vi "StateMachineExample.vi"() -> ()   [LabVIEW 2018]
doc: "Use this template to build a simple state machine design pattern. Each state executes code and determines which state to transition to."
panel:
  out "Data Ex out":T1
  in  "Data Ex":T1
  out "x .or. y?":bool
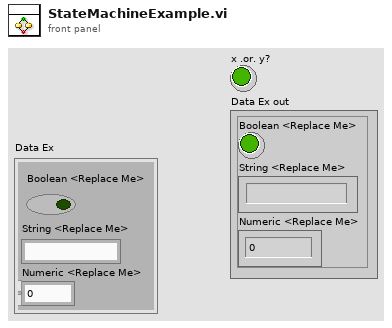
[diagram p1: front panel]
types:
  T1 = cluster{"Boolean <Replace Me>":bool, "String <Replace Me>":string, "Numeric <Replace Me>":dbl}
  T2 = enum16{"Initialize", "State 1", "State 2", "Exit"}
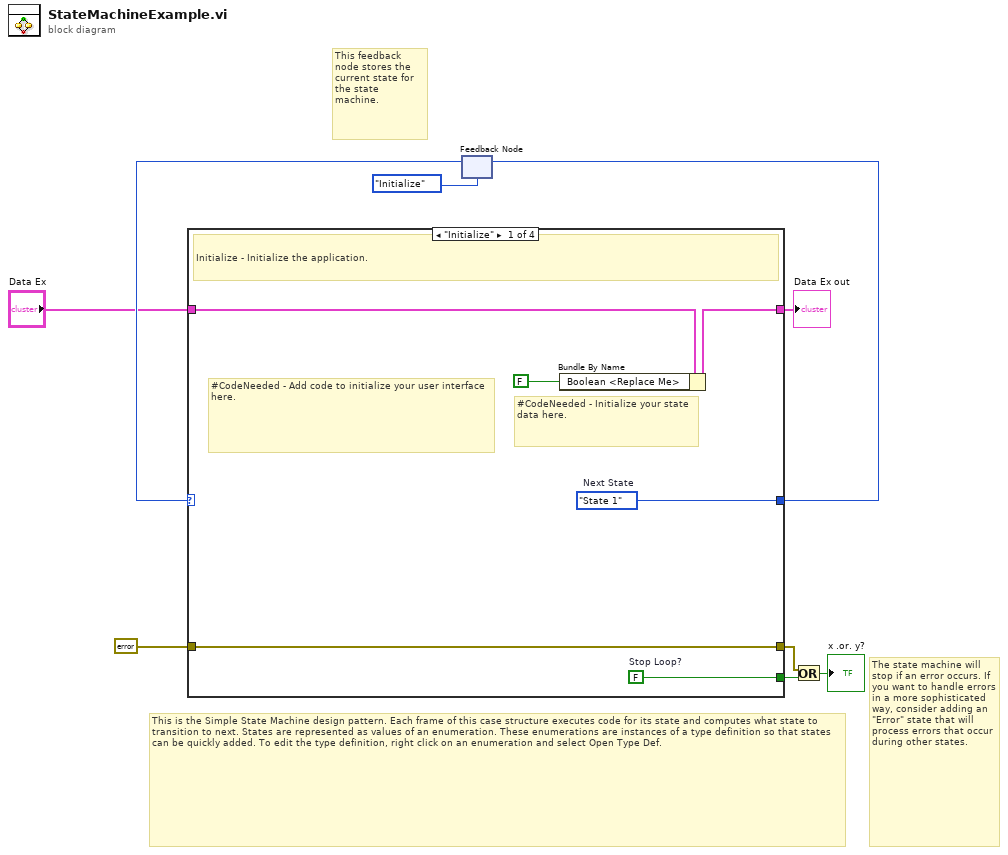
[diagram p0: block diagram]
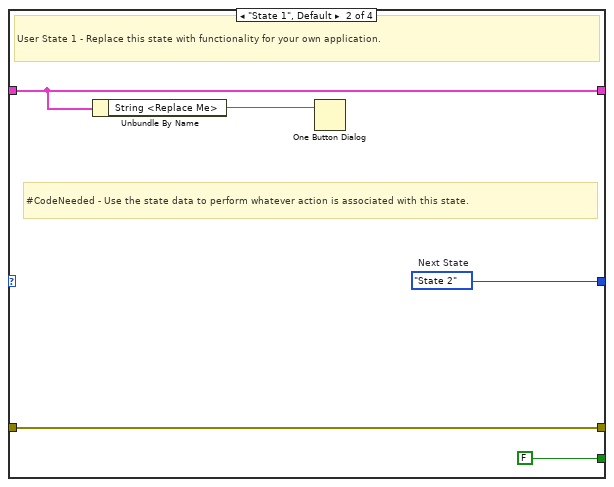
[diagram p2: hidden frame]
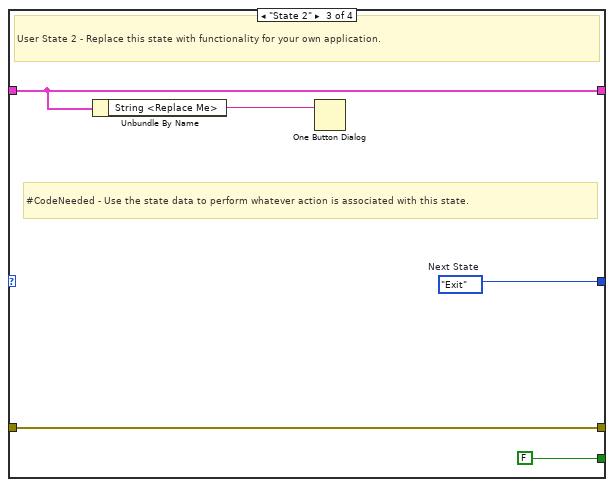
[diagram p3: hidden frame]
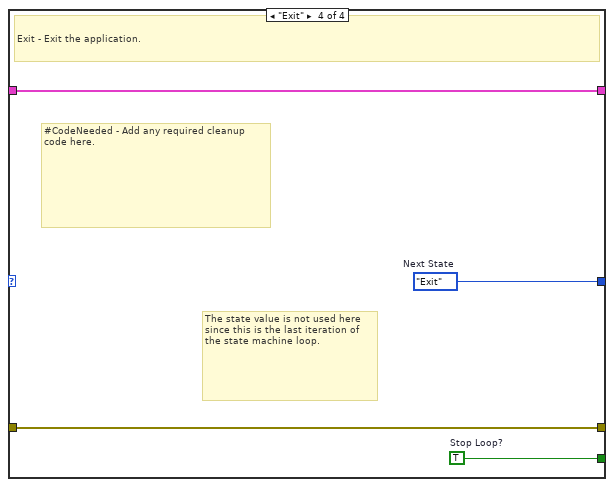
[diagram p4: hidden frame]
diagram:
  # "The state machine will stop if an error occurs. If you want to handle errors in a more sophisticated way, consider adding an \"Error\" state that will process errors that occur during other states."
  # "This feedback node stores the current state for the state machine."
  # "This is the Simple State Machine design pattern. Each frame of this case structure executes code for its state and computes what state to transition to next. States are represented as values of an enumeration. These enumerations are instances of a type definition so that states can be quickly added. To edit the type definition, right click on an enumeration and select Open Type Def."
  n1 = feedback #1(T2."Initialize" ("State")) -> (w3:T2)
  n2 = case shown="\"Initialize\"" w3 {
    tunnel: [w10 w16 w21 w26] -> w4
    tunnel: [w15 FALSE ("Stop Loop?") FALSE ("Stop Loop?") w28] -> w8
    tunnel: "Data Ex" -> [w14 w19 w24 w29]
    tunnel: [w13 w19 w24 w29] -> w1
    tunnel: errorcluster {"status"=FALSE, "code"=0, "source"=""} ("error constant") -> [w11 w17 w22 w27]
    tunnel: [w11 w17 w22 w27] -> w7
    frame "Initialize" {
      w10 = T2."State 1"  # Next State
      w15 = FALSE  # Stop Loop?
      # "#CodeNeeded - Initialize your state data here."
      # "#CodeNeeded - Add code to initialize your user interface here."
      # "Initialize - Initialize the application."
      n3 = Bundle By Name(cluster=w14, "Boolean <Replace Me>"=FALSE ("Replace_Me_Boolean")) -> (w13:T1)
    }
    frame "State 1", Default {
      w16 = T2."State 2"  # Next State
      # "#CodeNeeded - Use the state data to perform whatever action is associated with this state."
      # "User State 1 - Replace this state with functionality for your own application."
      n4 = Unbundle By Name(w19) -> ("String <Replace Me>"=w18:string)
      n5 = One Button Dialog(message=w18) -> ()  [unwired: 1 in, 1 out]
    }
    frame "State 2" {
      w21 = T2."Exit"  # Next State
      # "#CodeNeeded - Use the state data to perform whatever action is associated with this state."
      # "User State 2 - Replace this state with functionality for your own application."
      n6 = Unbundle By Name(w24) -> ("String <Replace Me>"=w23:string)
      n7 = One Button Dialog(message=w23) -> ()  [unwired: 1 in, 1 out]
    }
    frame "Exit" {
      w26 = T2."Exit"  # Next State
      w28 = TRUE  # Stop Loop?
      # "#CodeNeeded - Add any required cleanup code here."
      # "The state value is not used here since this is the last iteration of the state machine loop."
      # "Exit - Exit the application."
    }
  }
  "Data Ex out" <- w1
  n8 = feedback-in #1(w4) -> ()
  n9 = Or(x=w7, y=w8) -> (x .or. y?=→"x .or. y?":bool)
